vi "H-MEDI Error Popup.vi"(8 "error in (no error)":errorcluster caption="에러 입력(에러 없음)", 11 "Error Code Data In":string[][](array[string])) -> (0 "error out":errorcluster caption="에러 출력", 3 "Error Code Data Out":string[][](array[string]))   [LabVIEW 2019]
uses:
  <vilib>/Utility/miscctls.llb/LVRowAndColumnUnsignedTypeDef.ctl
panel:
  in  "Error List":i32(listbox)
  in  "Init":bool
  in  "Exit":bool
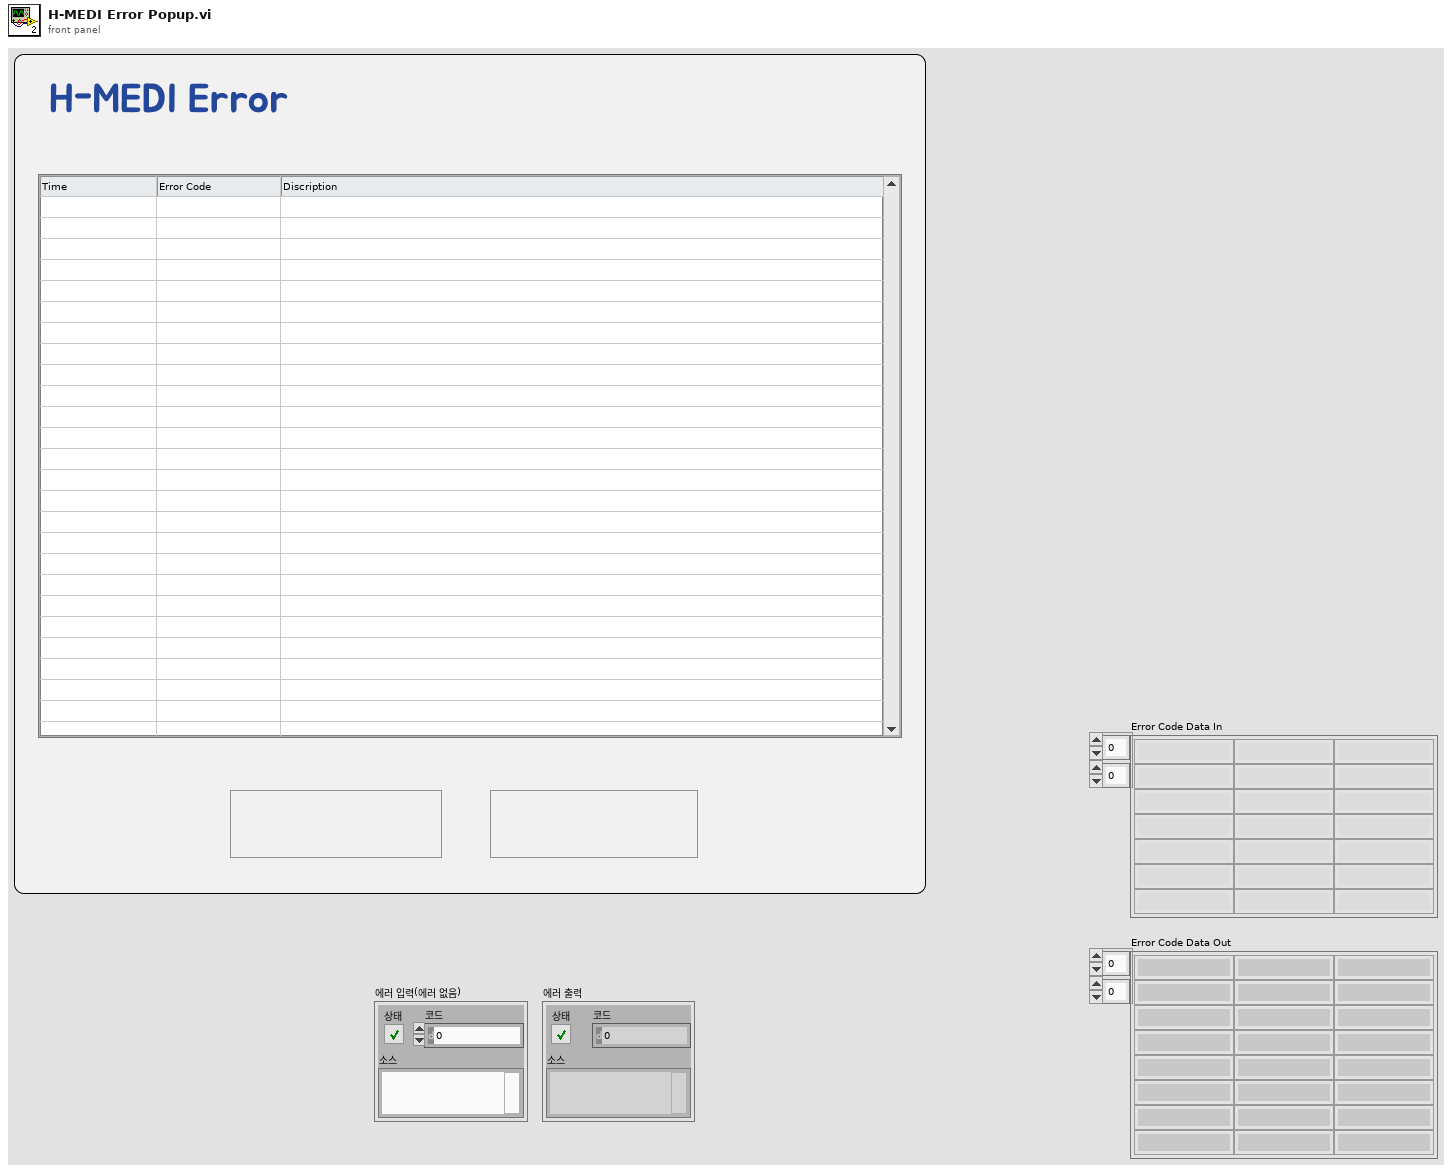
[diagram p1: front panel]
types:
  T1 = typedef "LVRowAndColumnUnsignedTypeDef.ctl" = cluster{"Row":u32, "Column":u32}
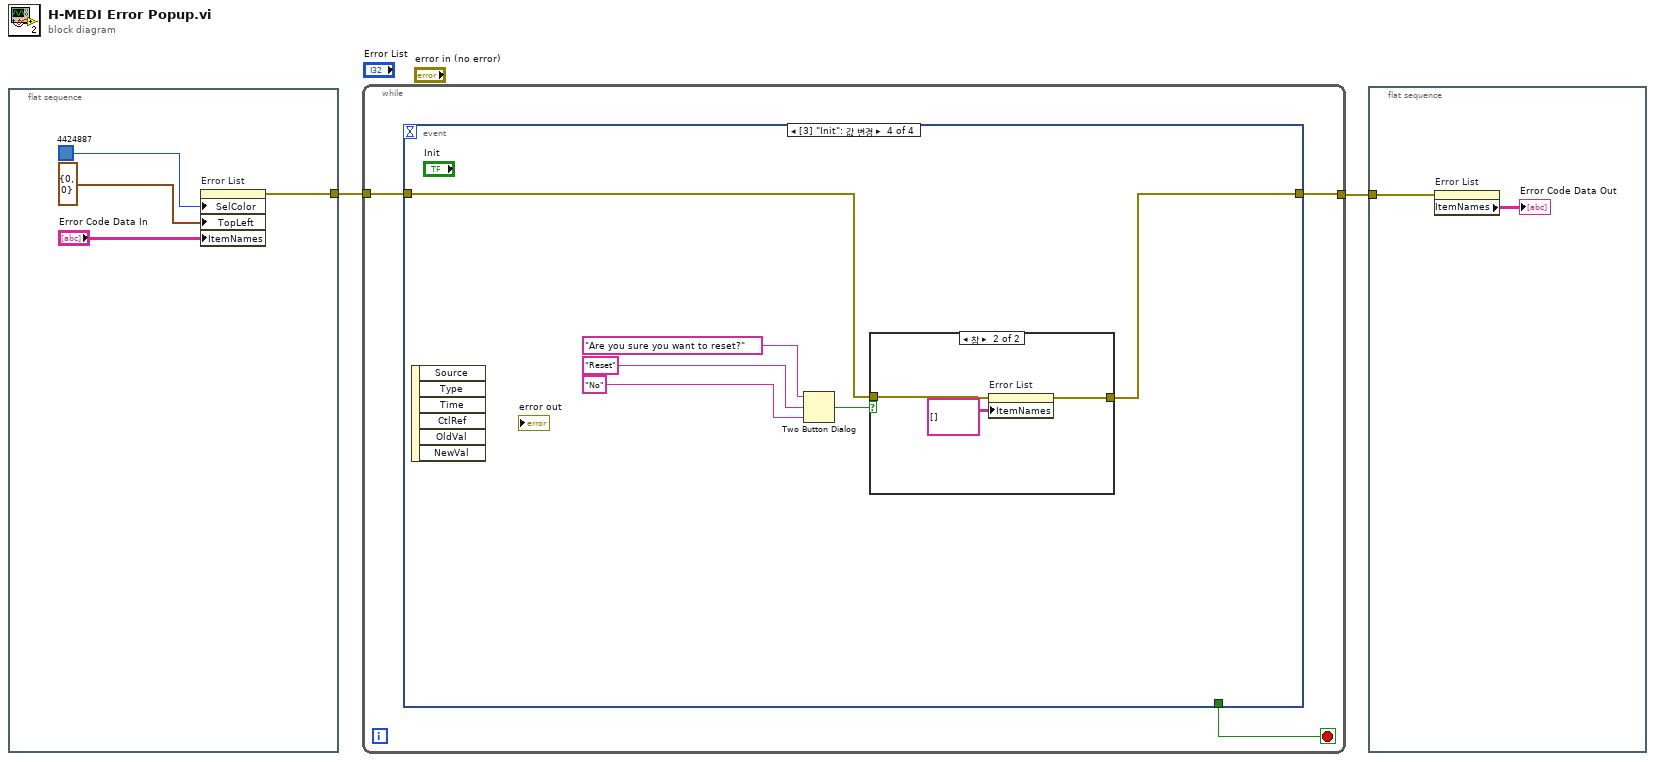
[diagram p0: block diagram]
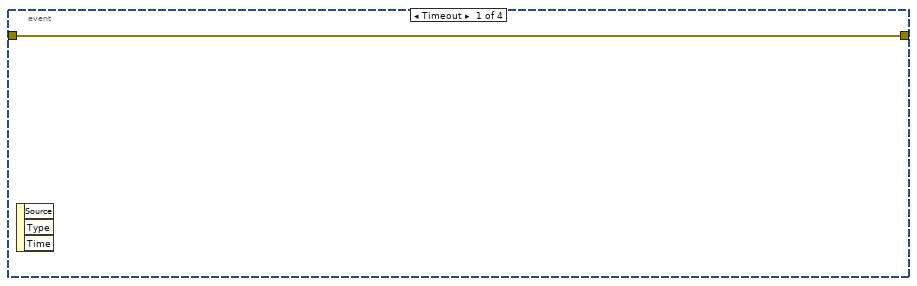
[diagram p2: hidden frame]
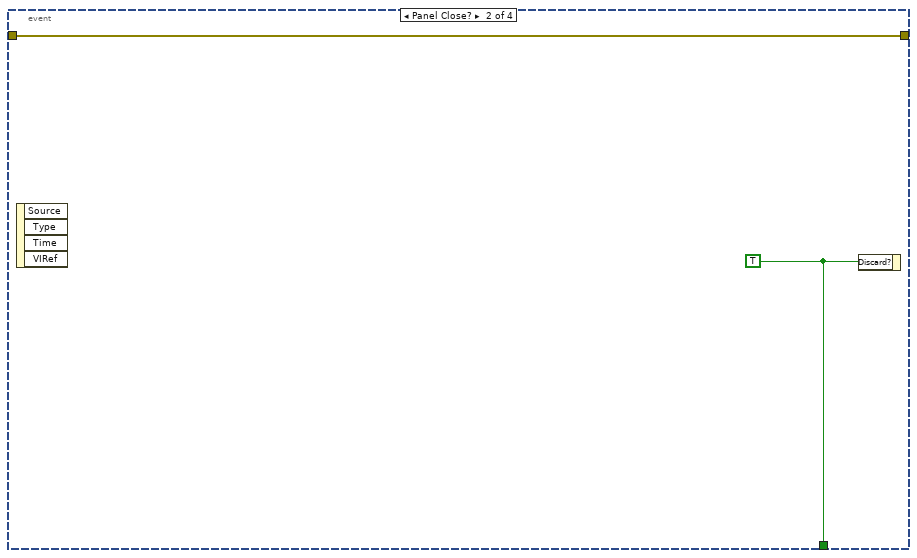
[diagram p3: hidden frame]
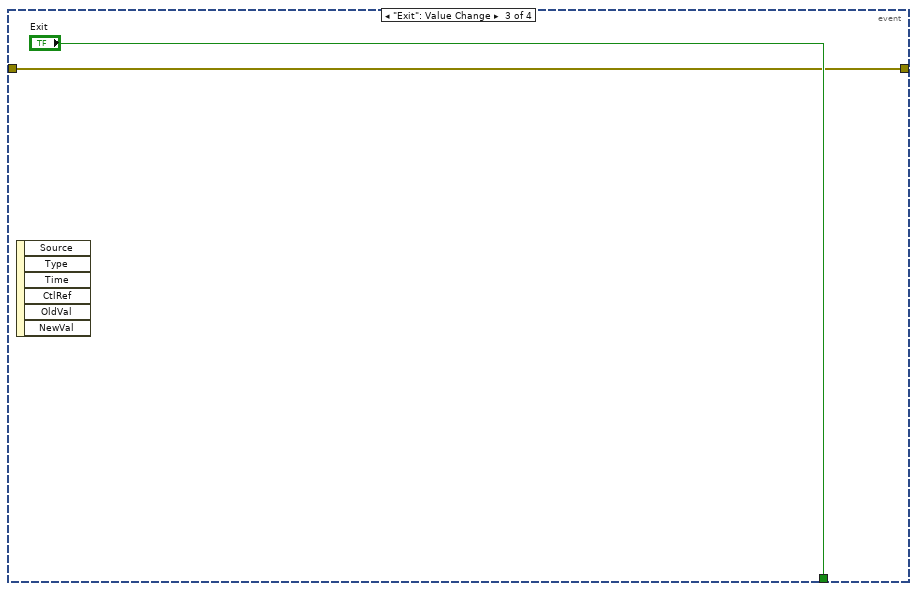
[diagram p4: hidden frame]
diagram:
  n1 = flat-sequence {
    tunnel: [w4] -> w2
    frame #0 {
      n2 = property on="Error List" class="MCListbox (엄격한)"("SelColor"=u32 4424887 ("선택 색"), "TopLeft"=T1 {"Row"=0, "Column"=0} ("왼쪽 위에 보이는 셀"), "ItemNames"="Error Code Data In") -> (error out=w4:errorcluster)  [unwired: 2 in, 1 out]
    }
  }
  n3 = while {
    tunnel: w2 -> [w8]
    tunnel: [w7] -> w1
    stop <- w9 stop-if-true
    n4 = event shown="[3] \"Init\": 값 변경" {
      selector: _ -> [_ _ _ _]
      dyn-events: _ -> [_ _ _ _]
      timeout: _ -> [_ _ _ _]
      tunnel: [_ w11 "Exit" _] -> w9
      tunnel: [w10 w12 w13 w15] -> w7
      tunnel: w8 -> [w10 w12 w13 w16]
      event Timeout {
        n5 = event-data() -> ()  [unwired: 1 in, 3 out]
      }
      event Panel Close? {
        w11 = TRUE
        n6 = event-data() -> ()  [unwired: 1 in, 4 out]
        n7 = event-data("Discard?"=w11) -> ()  [unwired: 1 in, 1 out]
      }
      event "Exit": Value Change {
        n8 = event-data() -> ()  [unwired: 1 in, 6 out]
      }
      event "Init": Value Change {
        n9 = event-data() -> ()  [unwired: 1 in, 6 out]
        n10 = Two Button Dialog(message="Are you sure you want to reset?" ("메시지"), 1:"No" ("거짓 버튼 이름(\"취소\")"), 2:"Reset" ("참 버튼 이름(\"확인\")")) -> (T button?=w20:bool)
        n11 = case shown="참" w20 {
          tunnel: w16 -> [w21 w23]
          tunnel: [w21 w22] -> w15
          frame False {
          }
          frame True {
            n12 = property on="Error List" class="MCListbox (엄격한)"(error in=w23, "ItemNames"=string[][] [] ("아이템 이름")) -> (error out=w22:errorcluster)  [unwired: 1 in, 1 out]
          }
        }
      }
    }
  }
  n13 = flat-sequence {
    tunnel: w1 -> [w26]
    frame #0 {
      n14 = property on="Error List" class="MCListbox (엄격한)"(error in=w26) -> ("ItemNames"=→"Error Code Data Out":string[][])  [unwired: 1 in, 2 out]
    }
  }
